vi "Crop to Bounding Box.vi"(8 "error in (no error)":errorcluster, 10 "Bounding Box":cluster{"x":sgl, "y":sgl}[](array[cluster]), 11 "Refnum in":T1) -> (0 "error out":errorcluster)   [LabVIEW 2012]
uses:
  <vilib>/vision/Image Controls.llb/IMAQ Image.ctl
  <vilib>/vision/NI_Vision_Development_Module.lvlib
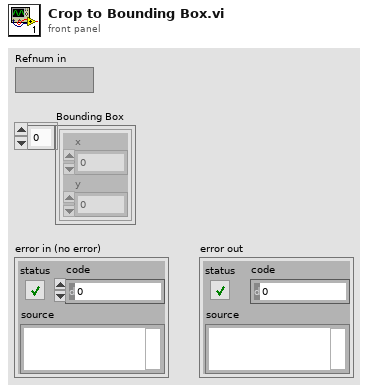
[diagram p1: front panel]
types:
  T1 = typedef "IMAQ Image.ctl" = refnum<image>
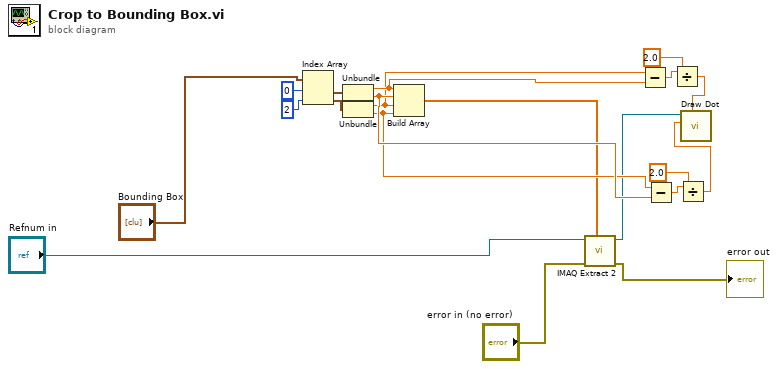
[diagram p0: block diagram]
diagram:
  n1 = Index Array(array="Bounding Box", index #1=0 ("index"), index #2=2 ("index")) -> (element #1=w4:cluster{"x":sgl, "y":sgl}, element #2=w5:cluster{"x":sgl, "y":sgl})
  n2 = Unbundle(w4) -> ("x"=w11:sgl, "y"=w19:sgl)
  n3 = Unbundle(w5) -> ("x"=w10:sgl, "y"=w18:sgl)
  n4 = Build Array(w11, w19, w10, w18) -> (w6:sgl[])
  n5 = call "IMAQ Extract 2"("Optional Rectangle"=w6, "error in (no error)"="error in (no error)", "Image Src"="Refnum in") -> ("error out"=→"error out":errorcluster, "Image Dst Out"=w9:T1)  [unwired: 7 in]
  n6 = Subtract(x=w10, y=w11) -> (x-y=w12:sgl)
  n7 = Subtract(x=w18, y=w19) -> (x-y=w16:sgl)
  n8 = Divide(x=w12, y=sgl 2.0) -> (x/y=w14:sgl)
  n9 = Divide(x=w16, y=sgl 2.0) -> (x/y=w20:sgl)
  n10 = call "Draw Dot.vi"("CenterX"=w14, "CenterY"=w20, "Refnum in"=w9) -> ()  [unwired: 7 in, 2 out]
